vi "SerializeTimeCalibration.vi"(10 "TimeCalibration in":string, 11 "cmd":enum16{"load", "save"}(ring)) -> (3 "TimeCalibration out":string)   [LabVIEW 2020]
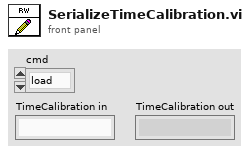
[diagram p1: front panel]
types:
  T1 = enum16{"open", "replace", "create", "open or create", "replace or create", "replace or create with confirmation"}
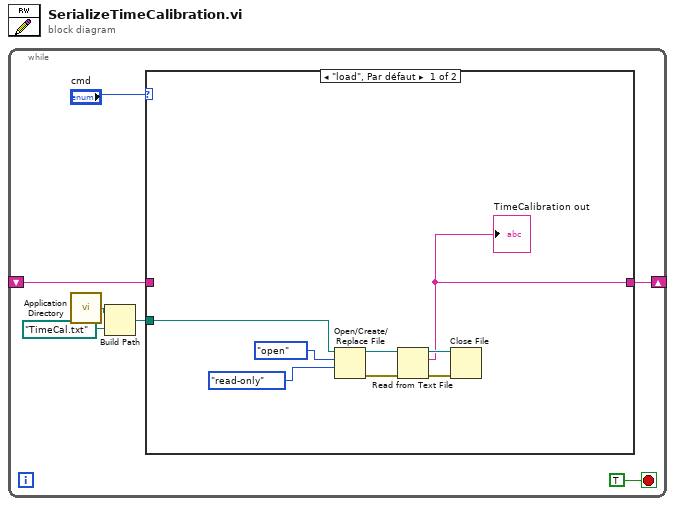
[diagram p0: block diagram]
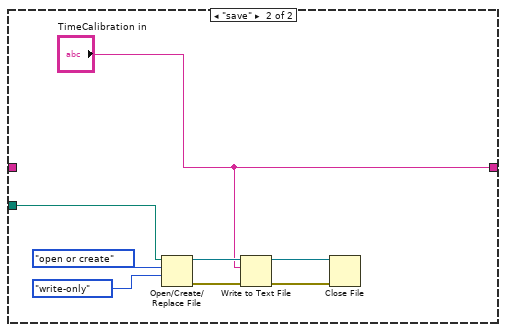
[diagram p2: hidden frame]
diagram:
  n1 = while {
    shift-right: [w5] -> _
    shift-left: _ -> [w4]
    stop <- TRUE stop-if-true
    n2 = call <vilib>:"Application Directory.vi"() -> ("Application Directory"=w3:path)
    n3 = Build Path(base path=w3, name or relative path=path "TimeCal.txt" ("chemin du fichier (utiliser une boîte de dialogue)")) -> (appended path=w1:path)
    n4 = case shown="\"load\", Par défaut" "cmd" {
      tunnel: [w9 "TimeCalibration in"] -> w5
      tunnel: w4 -> [_ _]
      tunnel: w1 -> [w8 w16]
      frame "load", Default {
        n5 = Open/Create/Replace File(file path (use dialog)=w8, operation (0:open)=T1."open" ("opération (0 : open)"), access (0:read/write)=enum16{"read/write", "read-only", "write-only"}."read-only" ("accès (0 : read/write)")) -> (refnum out=w10:refnum<file>, error out=w13:errorcluster)  [unwired: 3 in, 1 out]
        n6 = Read from Text File(file (use dialog)=w10, error in=w13) -> (refnum out=w11:refnum<file>, text=w9:string, error out=w12:errorcluster)  [unwired: 2 in, 1 out]
        "TimeCalibration out" <- w9
        n7 = Close File(refnum=w11, error in=w12) -> ()  [unwired: 2 out]
      }
      frame "save" {
        n8 = Open/Create/Replace File(file path (use dialog)=w16, operation (0:open)=T1."open or create" ("opération (0 : open)"), access (0:read/write)=enum16{"read/write", "read-only", "write-only"}."write-only" ("accès (0 : read/write)")) -> (refnum out=w21:refnum<file>, error out=w18:errorcluster)  [unwired: 3 in, 1 out]
        n9 = Write to Text File(file (use dialog)=w21, text="TimeCalibration in", error in=w18) -> (refnum out=w20:refnum<file>, error out=w17:errorcluster)  [unwired: 1 in, 1 out]
        n10 = Close File(refnum=w20, error in=w17) -> ()  [unwired: 2 out]
      }
    }
  }
